vi "ND_ArrayToNode(viaString).vi"(0 "Tree DVR in":refnum<data-value>, 1 "DBL Array":dbl[](array[numeric]), 3 "error in (no error)":errorcluster, 4 "NodePath":string) -> (5 "Tree DVR out":refnum<data-value>, 6 "TreeNode DVR out":refnum<data-value>, 7 "error out":errorcluster)   [LabVIEW 2014]
uses:
  <vilib>/MDSplus/Classes/Tree_Class/Tree.lvclass
  <vilib>/MDSplus/Classes/Data_Class/TreeNode_Class/TreeNode.lvclass
  <vilib>/MDSplus/Library/MDSplus.lvlib
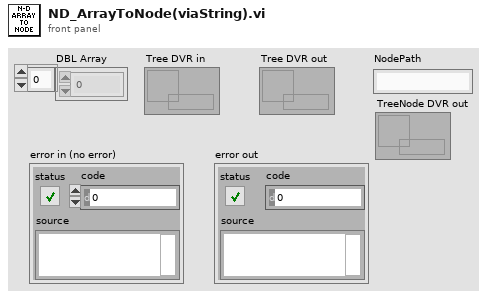
[diagram p1: front panel]
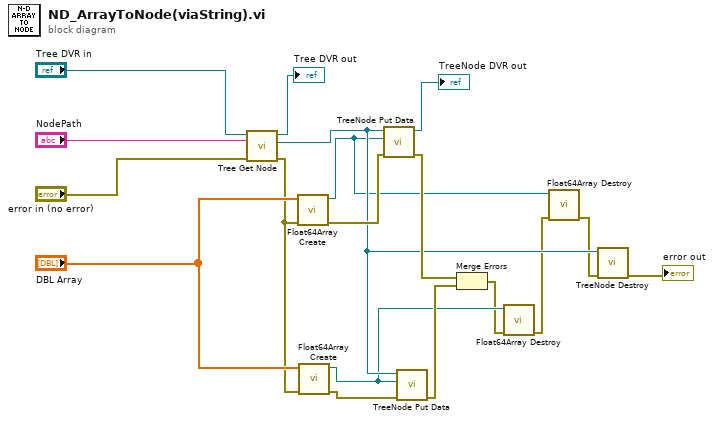
[diagram p0: block diagram]
diagram:
  n1 = call <vilib>:"Tree Get Node.vi"("error in (no error)"="error in (no error)", "Path"="NodePath", "Tree DVR in"="Tree DVR in") -> ("error out"=w11:errorcluster, "Node out"=w7:refnum<data-value>, "Tree DVR out"=→"Tree DVR out":refnum<data-value>)  [unwired: 6 in]
  n2 = call <vilib>:"Float64Array Create.vi"("error in (no error)"=w11, "DBL array in"="DBL Array") -> ("error out"=w14:errorcluster, "Float64Array DVR out"=w5:refnum<data-value>)  [unwired: 8 in]
  n3 = call <vilib>:"Float64Array Create.vi"("error in (no error)"=w11, "DBL array in"="DBL Array") -> ("error out"=w10:errorcluster, "Float64Array DVR out"=w6:refnum<data-value>)  [unwired: 8 in]
  n4 = call <vilib>:"TreeNode Put Data.vi"("error in (no error)"=w14, "Data"=w5, "TreeNode DVR in"=w7) -> ("error out"=w8:errorcluster, "TreeNode DVR out"=→"TreeNode DVR out":refnum<data-value>)  [unwired: 7 in]
  n5 = call <vilib>:"TreeNode Put Data.vi"("error in (no error)"=w10, "Data"=w6, "TreeNode DVR in"=w7) -> ("error out"=w9:errorcluster)  [unwired: 7 in, 1 out]
  n6 = Merge Errors(w8, w9) -> (w4:errorcluster)
  n7 = call <vilib>:"Float64Array Destroy.vi"("error in (no error)"=w4, "Float64Array DVR in"=w6) -> ("error out"=w3:errorcluster)  [unwired: 9 in]
  n8 = call <vilib>:"Float64Array Destroy.vi"("error in (no error)"=w3, "Float64Array DVR in"=w5) -> ("error out"=w2:errorcluster)  [unwired: 9 in]
  n9 = call <vilib>:"TreeNode Destroy.vi"("error in (no error)"=w2, "TreeNode DVR in"=w7) -> ("error out"=→"error out":errorcluster)  [unwired: 9 in]
